vi "PH_Cont-601k_PSU.evt call Set Voltage 0.vi"(0 "i ref in":refnum<vi>, 1 "Instance name":string="N/A", 5 "error in":errorcluster) -> (14 "i ref out":refnum<vi>, 19 "error out":errorcluster)   [LabVIEW 2014, in "PH_Cont-601k_PSU.lvlib"]
doc: "This VI calls an event by a simple call."
uses:
  PH_Cont-601k_PSU.lvlib
  CS_Core/CSSystem/CoreLib/CoreLib.short 2 byte array.vi
  CS_Core/BaseProcess/BaseProcess.lvlib
  CS_Core/CSSystem/CoreLib/CoreLib.lvlib
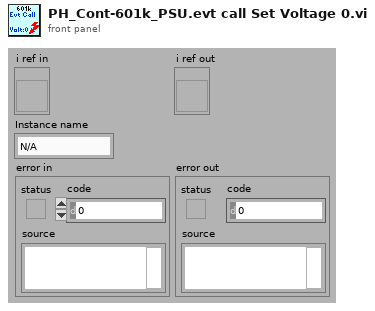
[diagram p1: front panel]
types:
  T1 = typedef "CoreDefs.rawDataType.ctl" = i8[]
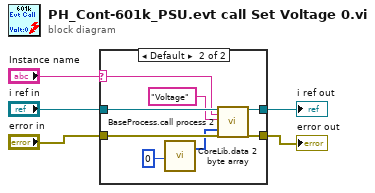
[diagram p0: block diagram]
diagram:
  n1 = case shown="Default" "Instance name" {
    selector: "Instance name" -> [_ w11]
    tunnel: [w6 w15] -> w1
    tunnel: "error in" -> [w6 w14]
    tunnel: [w7 w13] -> w2
    tunnel: "i ref in" -> [w7 w12]
    frame "", "N/A" {
    }
    frame Default {
      n2 = call-poly "CoreLib.data 2 byte array.vi"("i16"=i16 0 ("Value")) -> ("byteArray out"=w9:T1)  [unwired: 18 in]
      n3 = call "BaseProcess.call process 2.vi"("i ref in"=w12, "Object"=w11, "Selector"="Voltage", "Data"=w9, "error in (no error)"=w14) -> ("i ref out"=w13:refnum<vi>, "error out"=w15:errorcluster)  [unwired: 13 in]
    }
  }
  "error out" <- w1
  "i ref out" <- w2
